vi "colorUserItem Default--constant.vi"() -> (3 "default":string)   [LabVIEW 2021]
doc: "default list of user colors for the LabVIEW ini file"
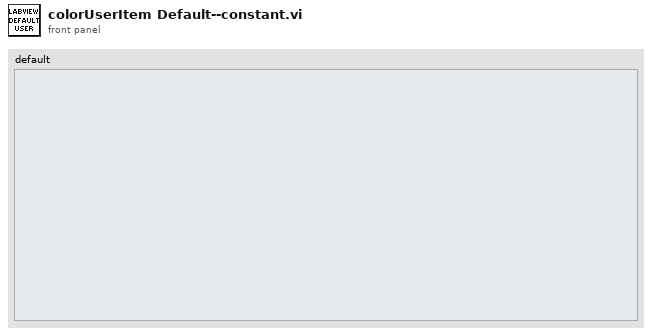
[diagram p1: front panel]
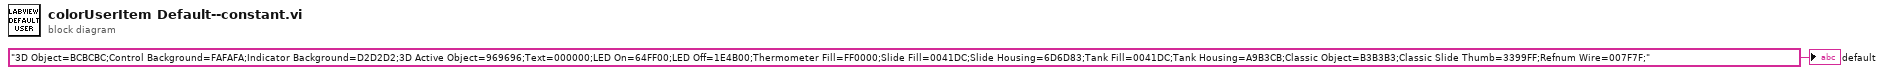
[diagram p0: block diagram]
diagram:
  "default" <- "3D Object=BCBCBC;Control Background=FAFAFA;Indicator Background=D2D2D2;3D Active Object=969696;Text=000000;LED On=64FF00;LED Off=1E4B00;Thermometer Fill=FF0000;Slide Fill=0041DC;Slide Housing=6D6D83;Tank Fill=0041DC;Tank Housing=A9B3CB;Classic Object=B3B3B3;Classic Slide Thumb=3399FF;Refnum Wire=007F7F;" ("default")
